vi "Convert Device Units to Acceleration (Polymorphic).vi"   [LabVIEW 2018, in "Zaber A Series.lvlib"]
doc: "Helper to convert device-specific units of acceleration to standard units.\n\nSelect a unit and enter an a device's acceleration quantity. The output will be the acceleration converted to the selected unit.\n\nIf you select a unit other than device units, you must also provide the Microstep Size conversion factor from microsteps to micrometers, which can be found in your device manual."
uses:
  Zaber A Series.lvlib
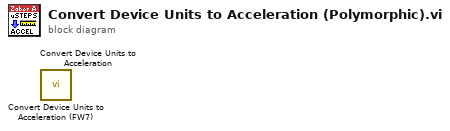
[diagram p0: block diagram]
diagram:
  n1 = call "Convert Device Units to Acceleration (FW7).vi"() -> ()  [unwired: 11 in, 1 out]
  n2 = call "Convert Device Units to Acceleration.vi"() -> ()  [unwired: 11 in, 1 out]
